vi "Start Main & OCU with Simulator.vi"() -> ()   [LabVIEW 2011]
doc: "Runs the main VI and the OCU on the same computer. simply here for ease of use."
uses:
  0-OCU/0 Typedefs/Maps.ctl
  2-Think/2 Typedefs/robot velocity.ctl
  0-OCU/0 Typedefs/Location of Think.ctl
  1,3 B-Simulation/1,3 B Typedefs/simulator bounds.ctl
  2-Think/2 Typedefs/Which Boat.ctl
  2-Think/2 Typedefs/eStopCommand.ctl
panel:
  in  "Robot Initial Position\nFrom Simulator SW corner":T1={"East"=20.0, "North"=20.0}
  in  "Map Name":T2="Lake Waban"
  # "running this VI will run OCU and Main on this computer."
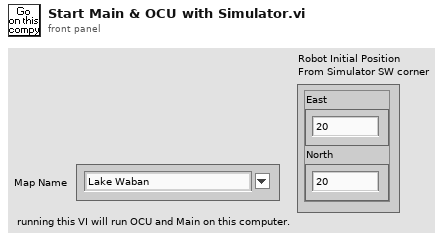
[diagram p1: front panel]
types:
  T1 = typedef "robot velocity.ctl" = cluster{"East":dbl, "North":dbl}
  T2 = typedef "Maps.ctl" = string
  T3 = typedef "eStopCommand.ctl" = enum16{"Reset E-Stop", "Get E-Stop", "Set E-Stop"}
  T4 = typedef "Image Type" = u32
  T5 = typedef "Which Boat.ctl" = enum16{"Competition Boat", "Small RC", "Simulation"}
  T6 = typedef "simulator bounds.ctl" = cluster{"Simulator E Range":dbl, "Simulator E Min":dbl, "Simulator N Range":dbl, "Simulator N Min":dbl}
  T7 = typedef "Location of Think.ctl" = string
  T8 = typedef "IMAQ Image.ctl" = refnum<image>
  T9 = typedef "0-Image Descriptor.ctl" = cluster{"Upper-Left Corner Coordinates":T10, "Meters/Pixel":dbl}
  T10 = typedef "UTM Location.ctl" = cluster{"UTM Zone":dbl, "Hemisphere":enum16{"North", "South"}, "East":dbl, "North":dbl}
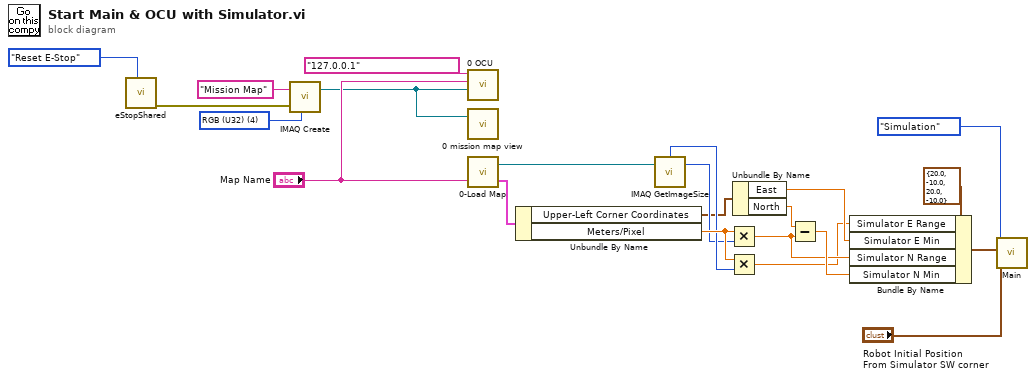
[diagram p0: block diagram]
diagram:
  w6 = T4 4 items=["Grayscale (U8)", "Grayscale (I16)", "Grayscale (SGL)", "Complex (CSG)", "RGB (U32)", "HSL (U32)", "RGB (U64)", "Grayscale (U16)"] ("Image Type")
  n1 = call "eStopShared.vi"("Command"=eStopCommand."Reset E-Stop") -> ("Error Out"=w3:errorcluster)  [unwired: 9 in, 1 out]
  n2 = call "IMAQ Create"("Image Name"="Mission Map", "Image Type"=w6, "error in (no error)"=w3) -> ("New Image"=w2:T8)  [unwired: 1 in, 2 out]
  n3 = call "0 OCU.vi"("Overview Image Ref In"=w2, "Map Name"="Map Name", "Location of THINK"=T7 "127.0.0.1") -> ()  [unwired: 9 in]
  n4 = call "0 mission map view.vi"("Image In"=w2) -> ()  [unwired: 3 in]
  n5 = call "0-Load Map.vi"("Map Name"="Map Name") -> ("Image Descriptor"=w21:T9, "Image Ref Out"=w20:T8)  [unwired: 1 in]
  n6 = Unbundle By Name(w21) -> ("Upper-Left Corner Coordinates"=w15:T10, "Meters/Pixel"=w19:dbl)
  n7 = call "IMAQ GetImageSize"("Image"=w20) -> ("Y Resolution"=w17:i32, "X Resolution"=w18:i32)  [unwired: 3 in, 1 out]
  n8 = Multiply(x=w19, y=w17) -> (x*y=w12:dbl)
  n9 = Multiply(x=w19, y=w18) -> (x*y=w10:dbl)
  n10 = Unbundle By Name(w15) -> ("East"=w11:dbl, "North"=w14:dbl)
  n11 = Subtract(x=w14, y=w12) -> (x-y=w13:dbl)
  n12 = Bundle By Name(cluster=T6 {"Simulator E Range"=20.0, "Simulator E Min"=-10.0, "Simulator N Range"=20.0, "Simulator N Min"=-10.0} ("Simulator Bounds"), "Simulator E Range"=w10, "Simulator E Min"=w11, "Simulator N Range"=w12, "Simulator N Min"=w13) -> (w9:T6)
  n13 = call "Main.vi"("Robot Initial Position\nFrom Simulator SW corner"="Robot Initial Position\nFrom Simulator SW corner", "Simulator Bounds"=w9, "Which Boat Am I?\n(unnecessary to set on RIO)"=Which_Boat."Simulation" ("Which Boat Am I?\n(unnecessary to set on RIO)")) -> ()  [unwired: 9 in]
